vi "FestoCPX.Station.Lamp.Blink.vi"(8 "error in (no error)":errorcluster) -> (0 "error out":errorcluster)   [LabVIEW 2016]
uses:
  FestoCPX.DO.Signal.ctl
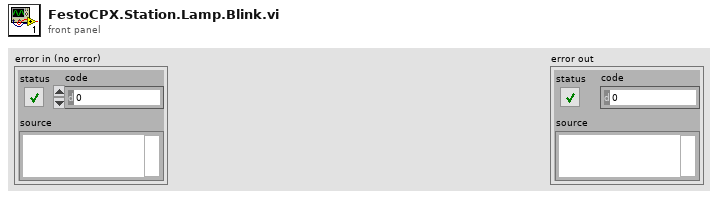
[diagram p1: front panel]
types:
  T1 = typedef "FestoCPX.DO.Signal.ctl" = enum16{"Safety Reset", "Air Main Valve", "Door Lock", "Button LED Start", "Button LED Stop", "Button LED Control", "Traffic LED Red", "Traffic LED Orange", "Traffic LED Green", "Horn", "Laser Interlock", "Laser Trigger", "Laser Fume Extractor", "Product Suction Gripper Slot 1 A", "Product Suction Gripper Slot 1 B", "Product Suction Gripper Slot 2 A", "Product Suction Gripper Slot 2 B", "Product Suction Gripper Slot 3 A", "Product Suction Gripper Slot 3 B", "Product Suction Gripper Slot 4 A", "Product Suction Gripper Slot 4 B", "Product Suction Gripper Final A", "Product Suction Gripper Final B", "Lamp", "Q1 Product Move Work", "Q1 Product Move Home", "Q2 Table Turn Work", "Q2 Table Turn Home", "Q3 Product Lift A", "Q3 Product Lift B", "Q4 Product Arm OK", "Q4 Product Arm NOK", "Q5 Product Arm Work", "Q6 Product BlowOut A", "Q6 Product BlowOut B"}
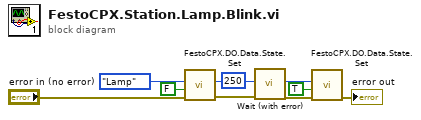
[diagram p0: block diagram]
diagram:
  w5 = FestoCPX.DO.Signal."Lamp"
  n1 = call "FestoCPX.DO.Data.State.Set.vi"("error in (no error)"="error in (no error)", "State"=FALSE, "CPX.DO"=w5) -> ("error out"=w7:errorcluster)  [unwired: 8 in]
  n2 = call "Wait (with error).vi"("error in (no error)"=w7, "milliseconds to wait"=u32 250) -> ("error out"=w6:errorcluster)  [unwired: 8 in, 1 out]
  n3 = call "FestoCPX.DO.Data.State.Set.vi"("error in (no error)"=w6, "State"=TRUE, "CPX.DO"=w5) -> ("error out"=→"error out":errorcluster)  [unwired: 8 in]
